vi "Make String Safe in Path.vi"(1 "replace string (\"\")":string, 2 "String In":string) -> (6 "Filesafe String Out":string)   [LabVIEW 2017]
doc: "Removes the characters that Windows does not allow in a file or folder name, so the result can be used inside a path. Wire replace string to substitute those characters instead of deleting them."
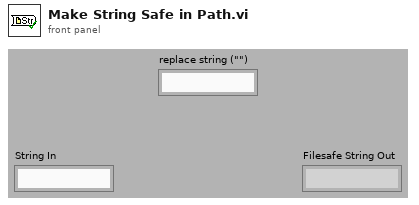
[diagram p1: front panel]
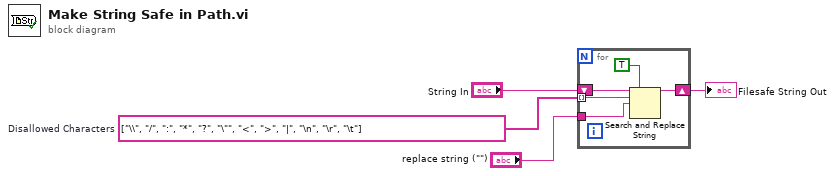
[diagram p0: block diagram]
diagram:
  w4 = string[] ["\\", "/", ":", "*", "?", "\"", "<", ">", "|", "\n", "\r", "\t"]  # Disallowed Characters
  n1 = for {
    tunnel: w4 -> [w7] mode=indexing
    shift-right: [w6] -> w2
    shift-left: "String In" -> [w8]
    tunnel: "replace string (\"\")" -> [w5]
    n2 = Search and Replace String(replace all?=TRUE ("replace all? (F)"), input string=w8, search string=w7, replace string=w5) -> (result string=w6:string)  [unwired: 4 in, 3 out]
  }
  "Filesafe String Out" <- w2
